vi "Do.vi"(8 "error in (no error)":errorcluster, 10 "Actor in":refnum<class "Actor.lvclass">, 11 "Test Dialog Return Msg":refnum<class "Test Dialog Return Msg.lvclass">) -> (0 "error out":errorcluster, 2 "Actor out":refnum<class "Actor.lvclass">)   [LabVIEW 2017, in "TopLevelApplication.lvlib" / "Test Dialog Return Msg.lvclass"]
doc: "(<B>Filename</B>: Actor Framework.lvlib:Message.lvclass:Do.vi)\n\nDefines what a message does when it is received by an actor. Generally, a message instructs an actor to invoke one of its methods. By default, this method does nothing. A child class must override it to define behavior. Create a child class by using the Actor Framework Message Maker dialog box.\n\n<License>\nCopyright © 2017 Composed Systems, LLC | All rights reserved\nwww.composed.io\n\nAuthor: Ethan Stern <ethan.stern@composed.io>\n\nThis software is provided \"AS IS\" WITHOUT WARRANTIES, either express or implied, AND IS FOR EDUCATIONAL PURPOSES ONLY.\n</License>"
uses:
  Test Dialog Return Msg.lvclass
  <vilib>/ActorFramework/Actor/Actor.lvclass
  ConcreteViewModel/ConcreteViewModel.lvclass
  C:/Program Files (x86)/National Instruments/LabVIEW 2017/vi.lib/ActorFramework/Actor/Actor.lvclass
  Test Dialog Return Msg.lvclass/Test Dialog Return Msg.ctl
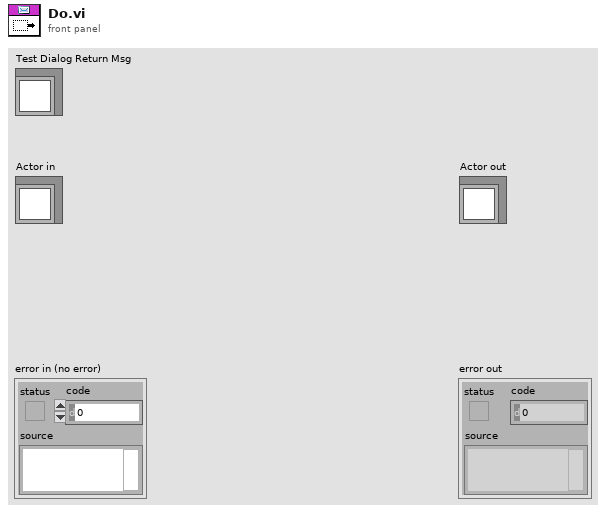
[diagram p1: front panel]
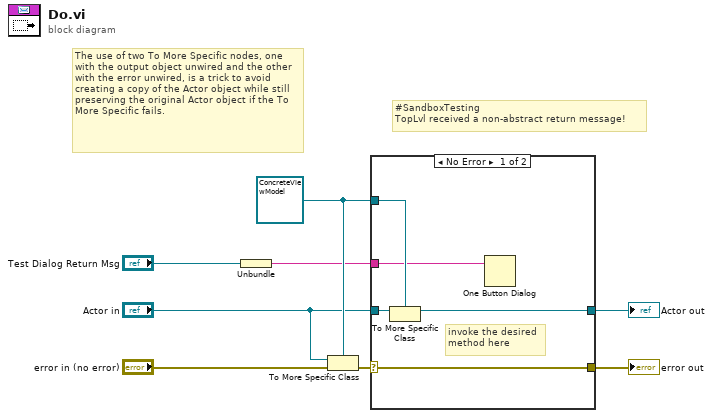
[diagram p0: block diagram]
diagram:
  w8 = refnum<class "ConcreteViewModel.lvclass"> refnum ("Actor in")
  # "#SandboxTesting\nTopLvl received a non-abstract return message!"
  # "The use of two To More Specific nodes, one with the output object unwired and the other with the error unwired, is a trick to avoid creating a copy of the Actor object while still preserving the original Actor object if the To More Specific fails."
  n1 = Unbundle("Test Dialog Return Msg") -> (w1:string)
  n2 = To More Specific Class(target class=w8, reference="Actor in", error in="error in (no error)") -> (error out=w7:errorcluster)  [unwired: 1 out]
  n3 = case shown="No Error" w7 {
    selector: w7 -> [w10 w15]
    tunnel: [w10 w15] -> w5
    tunnel: [w11 w14] -> w3
    tunnel: "Actor in" -> [w13 w14]
    tunnel: w8 -> [w12 _]
    tunnel: w1 -> [w9 _]
    frame No Error {
      # "invoke the desired\nmethod here"
      n4 = To More Specific Class(target class=w12, reference=w13) -> (specific class reference=w11:refnum<class "ConcreteViewModel.lvclass">)  [unwired: 1 in, 1 out]
      n5 = One Button Dialog(message=w9) -> ()  [unwired: 1 in, 1 out]
    }
    frame Error {
      # "If type check fails, pass the original object out again."
    }
  }
  "error out" <- w5
  "Actor out" <- w3
